vi "Receiver_Example - 2 Channel - Experiment_8.vi"() -> ()   [LabVIEW 2022 SP3]
uses:
  <vilib>/httpClient/LabVIEWHTTPClient.lvlib
panel:
  out "Boolean 7":bool
  out "HP - CH0":dbl format="%#_4g"
  out "Numeric":i32
  out "Boolean 6":bool
  out "Boolean 5":bool
  in  "url":string="http://Cobot280-01.local:5000"
  out "x = 0?":bool
  out "iterationsIM":dbl
  in  "State":i32
  in  "Counter":dbl
  in  "OFDM - 4QAM/16QAM":bool
  in  "Tab Control 3":enum32{"OFDM - 4QAM", "16QAM"}(tab)
  in  "Tab Control":enum32{"USRP Parameters", "Rx Info", "BER"}(tab)
  in  "USRP ControledParameters":T1={"Active Antenna"="RX2", "Gain (dB)"=10.0, "Carrier Frequency"=2400000000.0, "IQ Rate"=2000000.0, "Active channels"="0,1"} {"IQ Rate" format="%#_6p"; "Carrier Frequency" format="%#_6p"; "Gain (dB)" format="%#_6f"}
  in  "Device selection":refnum<k15>="RIO0"
  in  "Trigger level":dbl=0.005 format="%f"
  out "CH0":T2
  out "CH1":T2
  out "SIG valid? - CH1":bool
  out "SIG valid? - CH0":bool
  out "Frequency offset - CH1":dbl
  out "Frequency offset - CH0":dbl
  out "Coerced Parameters":T3={"IQ Rate"=100000.0, "Carrier  Freq."=100000.0, "Gain"=0.0} {"Gain" format="%#_6f"; "Carrier  Freq." format="%#_6p"; "IQ Rate" format="%#_6p"}
  out "Error out":errorcluster
  in  "Expected message LP - CH0":string="Non Critical Data\nNon Critical Data\nNon Critical Data\nNon Critical Data\nNon Critical Data"
  in  "Expected message - CH1":string="Critical Dataaaaa\nCritical Dataaaaa\nCritical Dataaaaa\nCritical Dataaaaa\nCritical Dataaaaa"
  out "Expected message LP Detected CH0":string="Non Critical Data\nNon Critical Data\nNon Critical Data\nNon Critical Data\nNon Critical Data"
  out "Expected message HP Detected CH1":string="Non Critical Data\nNon Critical Data\nNon Critical Data\nNon Critical Data\nNon Critical Data"
  in  "Boolean":bool
  in  "Boolean 3":bool
  out "Expected message HP Detected CH0":string="Non Critical Data\nNon Critical Data\nNon Critical Data\nNon Critical Data\nNon Critical Data"
  in  "Expected message HP - CH0":string="Critical Dataaaaa\nCritical Dataaaaa\nCritical Dataaaaa\nCritical Dataaaaa\nCritical Dataaaaa"
  in  "Boolean 2":bool
  out "Inst. BER HP - CH0":dbl format="%#_4g"
  out "Acc. BER HP - CH0":dbl format="%#_4g"
  out "Acum. Err HP - CH0":dbl
  out "No. Bits HP - CH0":dbl
  out "Acc. BER LP - CH0":dbl format="%#_4g"
  out "Inst. BER - CH1":dbl format="%#_4g"
  out "Inst. BER LP - CH0":dbl format="%#_4g"
  out "No. Bits - CH1":dbl
  out "No. Bits LP - CH0":dbl
  out "Acum. Err - CH1":dbl
  out "Acum. Err LP - CH0":dbl
  in  "Record BER":bool
  in  "Refresh Button":bool
  out "Acc. BER - CH1":dbl format="%#_4g"
  in  "Low-Power Window Size - CH0":dbl=15.0 format="%#_6p"
  in  "High-Power Window Size":dbl=15.0 format="%#_6p"
  in  "Tab Control 2":enum32{"1 Channel", "2 Channel"}(tab)
  in  "Save data 1 channel":bool
  out "Constellation Map 1 Channel":cdb[](graph)
  out "Low-Power BER - 1 Channel":dbl(graph)
  out "High-Power BER - 1 Channel":dbl(graph)
  out "High-Power Decoded message - 1 Channel":string
  out "Low-Power Decoded message - 1 Channel":string
  out "Low-Power Decoded message - CH0":string
  out "Decoded message - CH1":string
  out "Constellation Map 2 Channel":cluster{"Constellation":cdb[]}[](graph)
  out "Low-Power BER - CH0":dbl(graph)
  out "High-Power BER":T4(graph)
  out "High-Power Decoded message - CH0":string
  out "CH1 2":bool
  out "CH0 2":bool
  in  "Save data 2 channels":bool
  in  "Channel":bool
  in  "Save data":bool
  out "Expected message  HP  Detected 2":string="Critical Dataaaaa\nCritical Dataaaaa\nCritical Dataaaaa\nCritical Dataaaaa\nCritical Dataaaaa"
  in  "Boolean 4":bool
  in  "High-Power Window Size 2":dbl=15.0 format="%#_6p"
  out "High-Power Instantaneous BER Graph 2":u8(slide) scale=0.0..100.0
  out "High-Power BER Graph 2":dbl(graph)
  out "No. Bits HP 2":dbl
  out "Acc. BER  HP 2":dbl format="%#_4g"
  out "Acum. Err HP 2":dbl
  out "Inst. BER HP 2":dbl format="%#_4g"
  in  "Expected message 2 HP 2":string="Critical Dataaaaa\nCritical Dataaaaa\nCritical Dataaaaa\nCritical Dataaaaa\nCritical Dataaaaa"
  out "High-Power Decoded Message 2":string
  in  "Record BER 2":bool
  out "Constellation Map 2":cdb[](graph)
  out "Frequency offset 2":dbl
  out "SIG valid? 2":bool
  in  "Refresh Button 2":bool
  out "Error out 2":errorcluster
  in  "error in (no error)":errorcluster
  # "OFDM Superposition Coded Receiver"
  # "1 Channel"
  # "2 Channel"
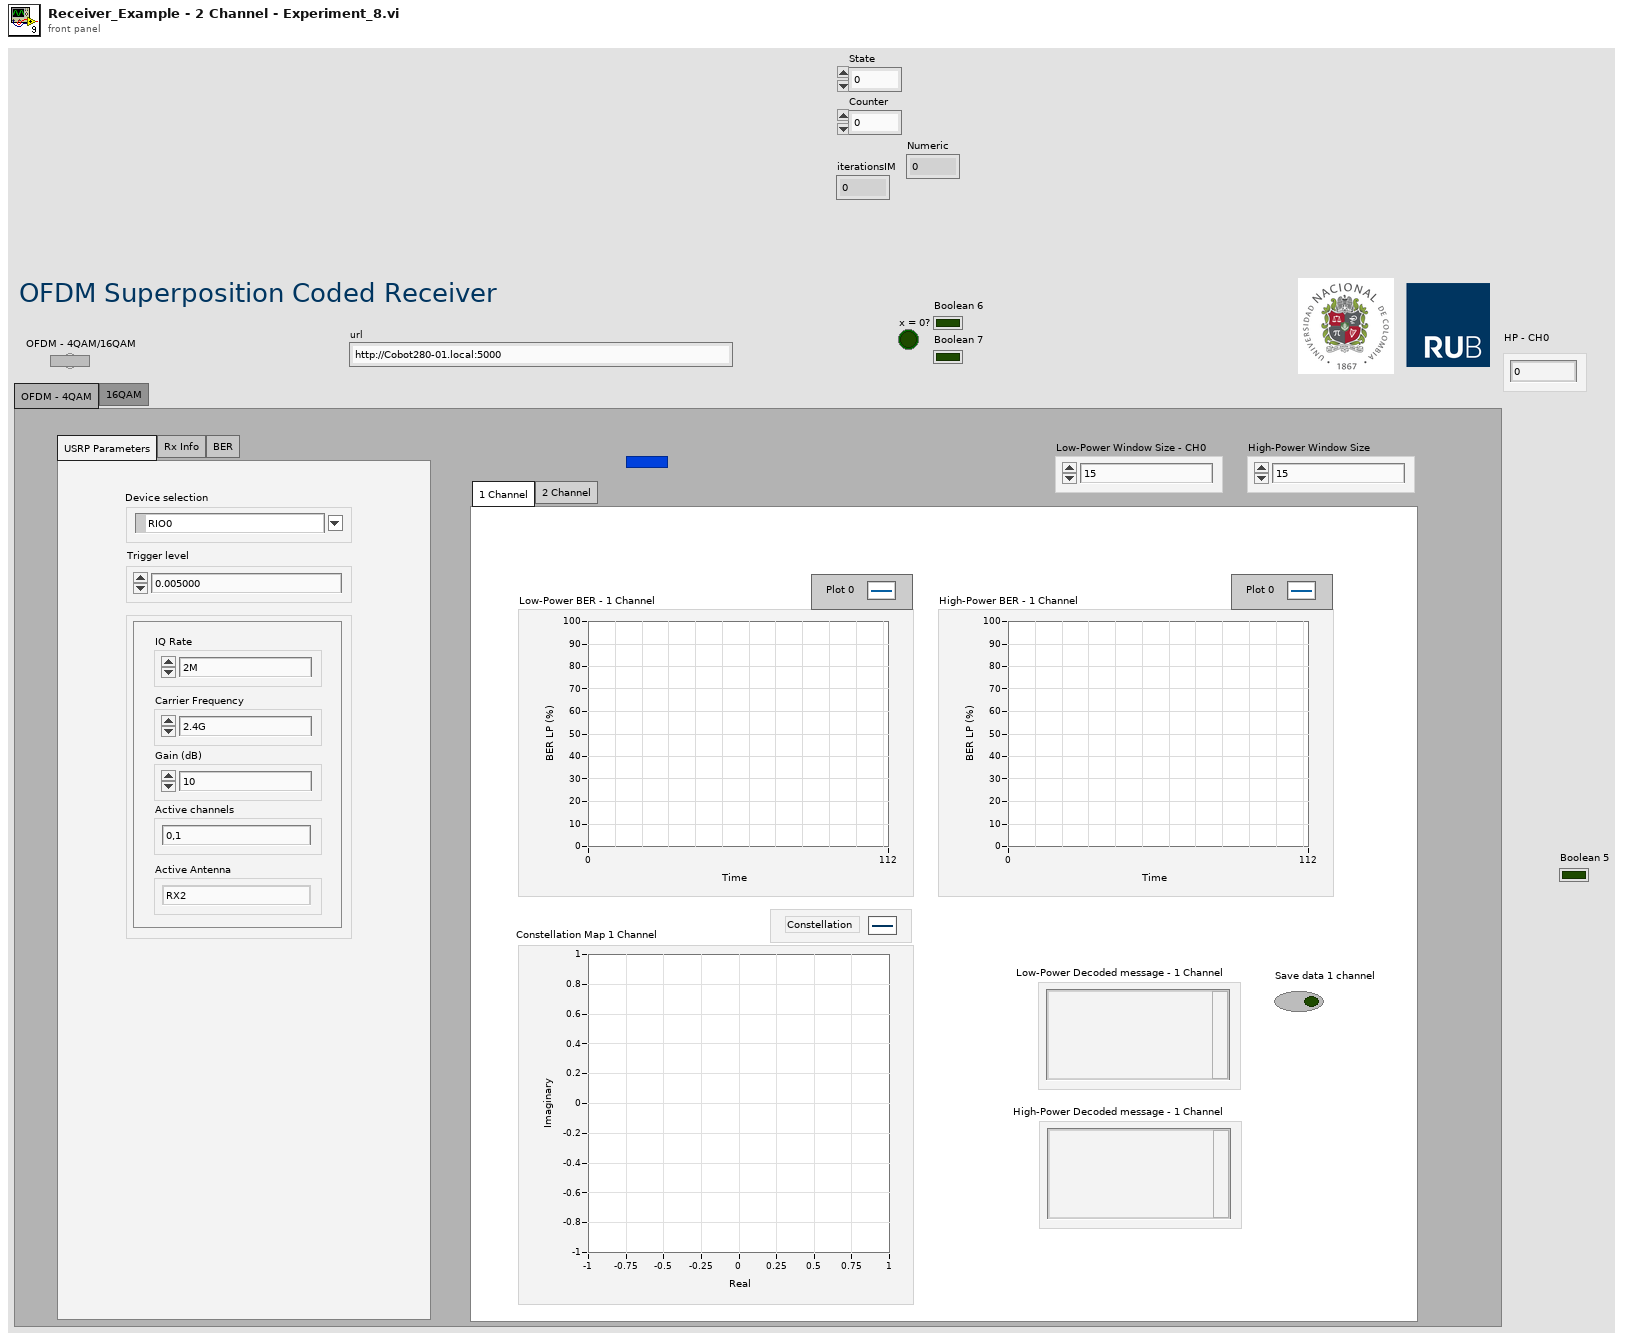
[diagram p1: front panel]
types:
  T1 = cluster{"Active Antenna":string, "Gain (dB)":dbl, "Carrier Frequency":dbl, "IQ Rate":dbl, "Active channels":string}
  T2 = cluster{"Modulation type":enum16{"QPSK(4QAM)", "64QAM", "16QAM", "BPSK"}, "BCC rate (k/n)":enum16{"1/2", "2/3", "3/4"}}
  T3 = cluster{"IQ Rate":dbl, "Carrier  Freq.":dbl, "Gain":dbl}
  T4 = cluster{"Graph Instantaneous BER":dbl, "Graph Instantaneous BER":dbl, "Inst. BER - CH1":dbl}
  T5 = enum16{"open", "replace", "create", "open or create", "replace or create", "replace or create with confirmation"}
  T6 = typedef "LabVIEWHTTPClient.lvlib/ClientHandle.ctl" = refnum<k1>
  T7 = typedef "angle_speed_def.ctl" = cluster{"degrees":dbl[], "speed":i32}
  T8 = cluster{"coerced IQ rate":dbl, "coerced carrier frequency":dbl, "coerced gain":dbl}
  T9 = cluster{"Graph Instantaneous BER":dbl, "Graph Instantaneous BER":dbl, "Graph Instantaneous BER":dbl}
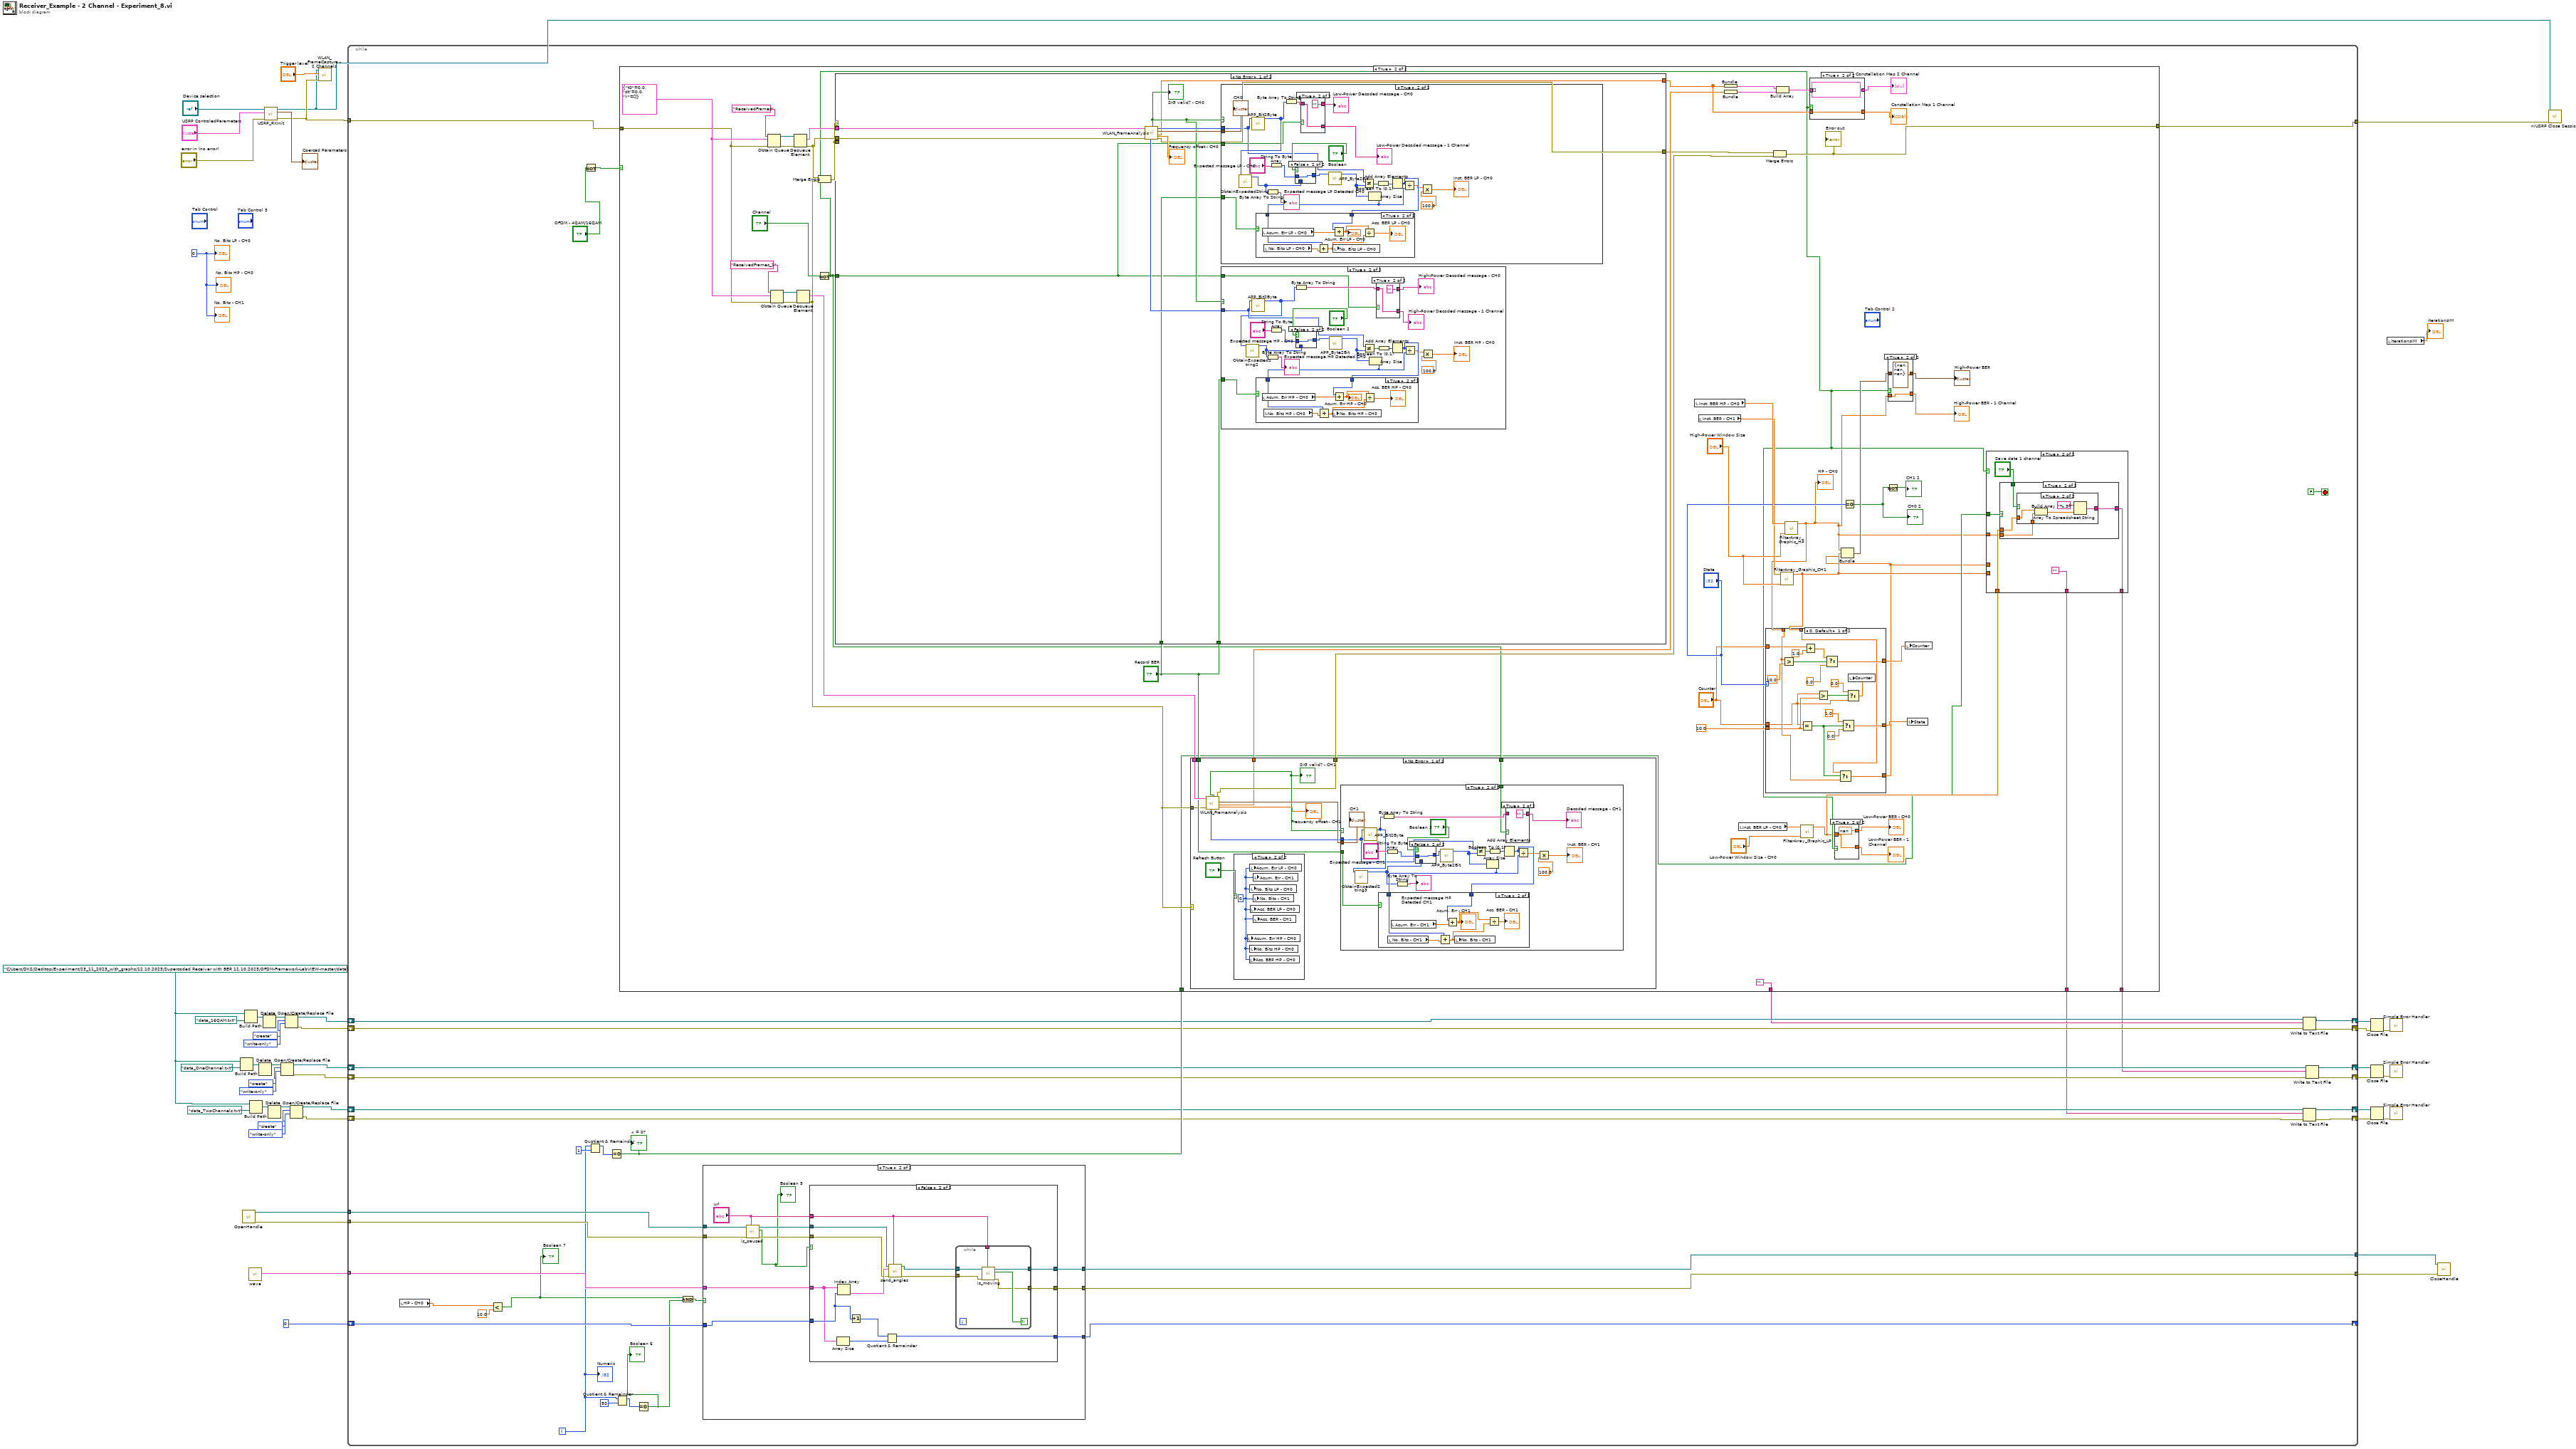
[diagram p0: block diagram]
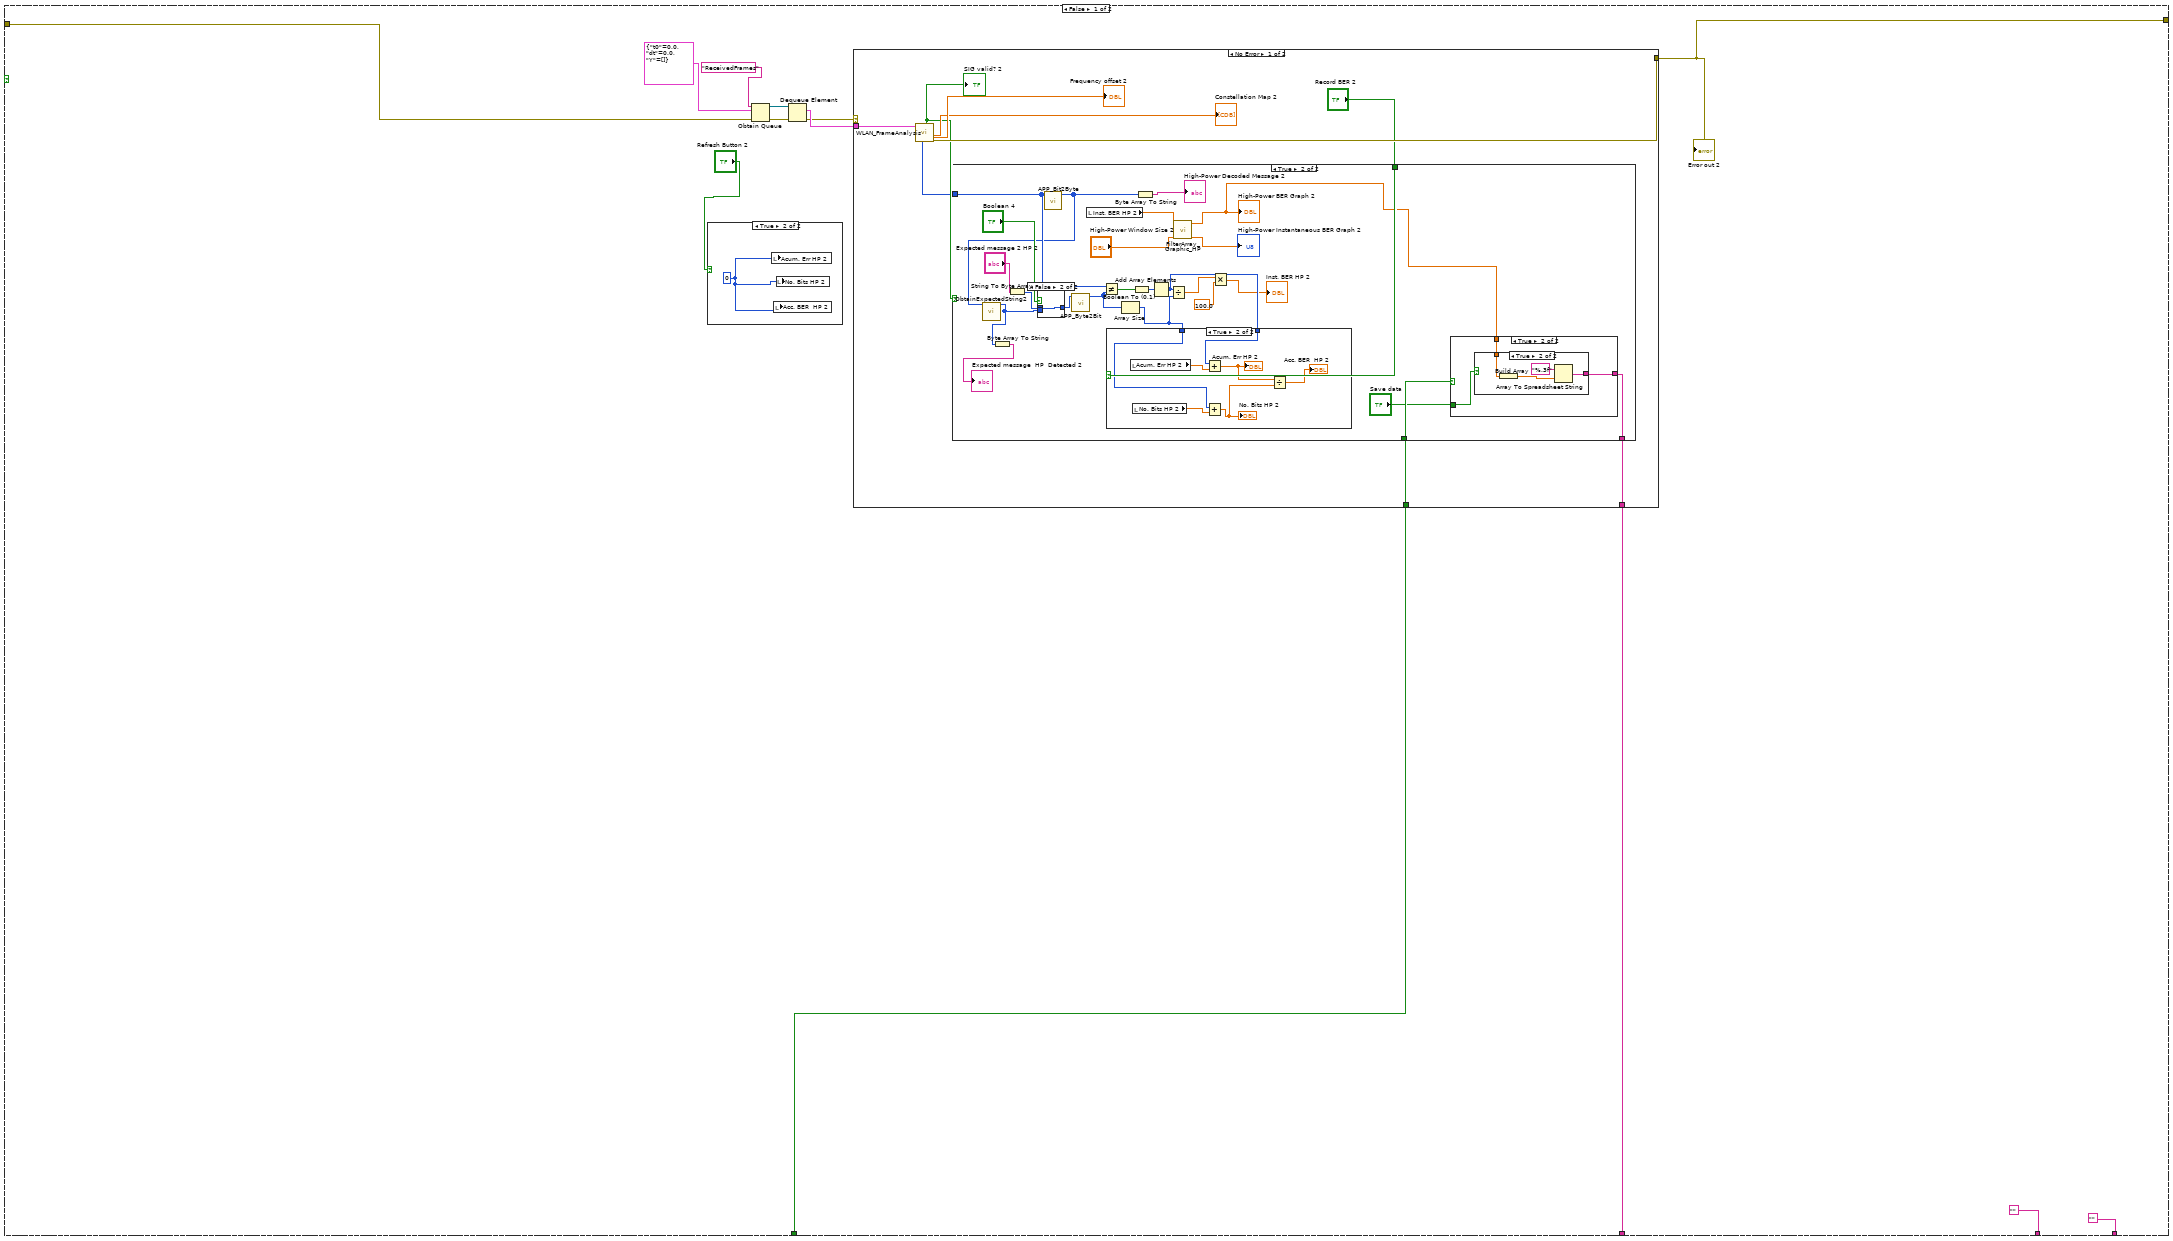
[diagram p4: hidden frame]
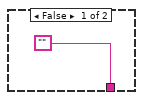
[diagram p6: hidden frame]
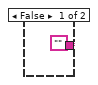
[diagram p7: hidden frame]
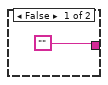
[diagram p8: hidden frame]
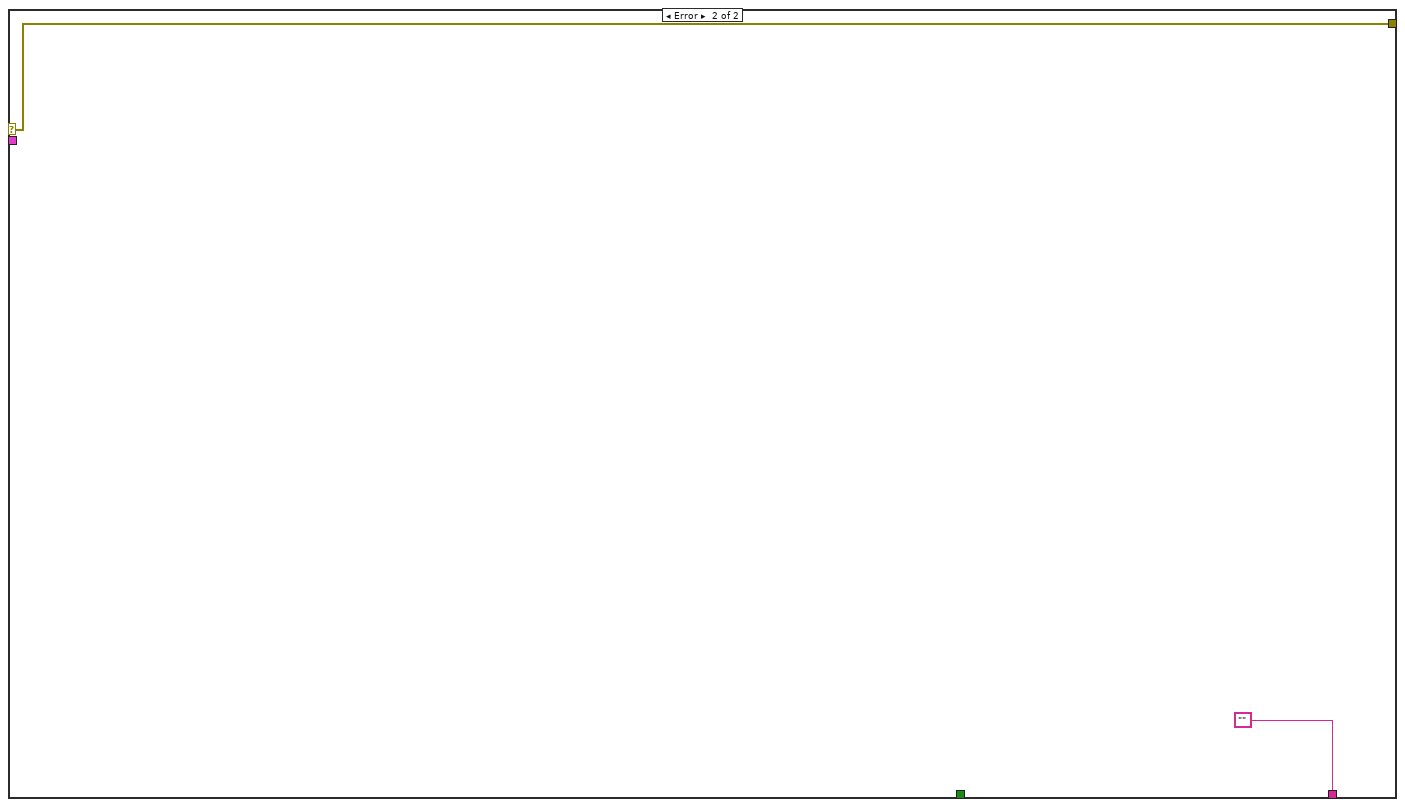
[diagram p11: hidden frame]
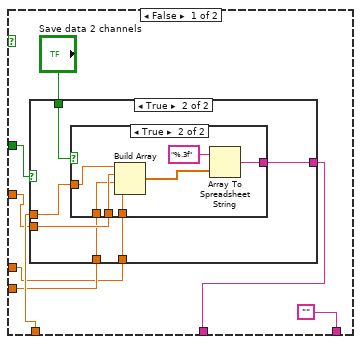
[diagram p12: hidden frame]
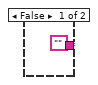
[diagram p13: hidden frame]
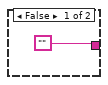
[diagram p14: hidden frame]
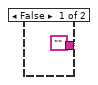
[diagram p15: hidden frame]
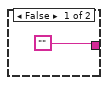
[diagram p16: hidden frame]
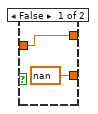
[diagram p17: hidden frame]
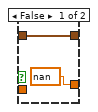
[diagram p18: hidden frame]
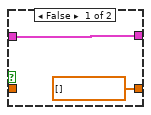
[diagram p19: hidden frame]
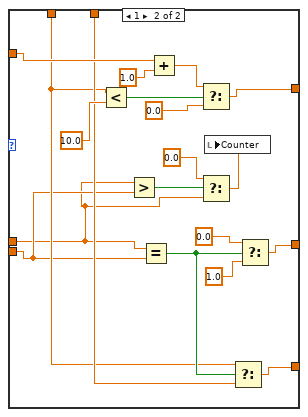
[diagram p20: hidden frame]
diagram:
  w17 = path "C:/Users/DKS/Desktop/Experiment/23_11_2023_with_graphs/12.10.2023/Supercoded Receiver with BER 12.10.2023/OFDM-Framework-LabVIEW-master/data"
  w39 = 0
  n1 = Build Path(base path=w17, name or relative path=path "data_OneChannel.txt" ("default name")) -> (appended path=w27:path)
  n2 = call <vilib>:"OpenHandle.vi"() -> ("client handle out"=w6:T6, "error out"=w5:errorcluster)  [unwired: 14 in]
  n3 = Build Path(base path=w17, name or relative path=path "data_16QAM.txt" ("default name")) -> (appended path=w37:path)
  n4 = call "wave.vi"() -> ("sequenz"=w4:T7[])  [unwired: 11 in]
  n5 = Build Path(base path=w17, name or relative path=path "data_TwoChannels.txt" ("default name")) -> (appended path=w22:path)
  n6 = Delete(path (use dialog)=w27) -> (deleted path=w26:path)  [unwired: 4 in, 2 out]
  n7 = Delete(path (use dialog)=w37) -> (deleted path=w36:path)  [unwired: 4 in, 2 out]
  n8 = call "USRP_RXInit.vi"("device names"="Device selection", "USRP ControledParameters"="USRP ControledParameters", "error in (no error)"="error in (no error)") -> ("session handle out"=w42:refnum<k15>, "USRP CoercedParamters"=→"Coerced Parameters":T8, "error out"=w45:errorcluster)  [unwired: 5 in]
  n9 = Delete(path (use dialog)=w22) -> (deleted path=w21:path)  [unwired: 4 in, 2 out]
  n10 = Open/Create/Replace File(file path (use dialog)=w26, operation (0:open)=T5."create", access (0:read/write)=enum16{"read/write", "read-only", "write-only"}."write-only") -> (refnum out=w14:refnum<file>, error out=w13:errorcluster)  [unwired: 1 in, 3 out]
  n11 = Open/Create/Replace File(file path (use dialog)=w36, operation (0:open)=T5."create", access (0:read/write)=enum16{"read/write", "read-only", "write-only"}."write-only") -> (refnum out=w30:refnum<file>, error out=w31:errorcluster)  [unwired: 1 in, 3 out]
  n12 = Open/Create/Replace File(file path (use dialog)=w21, operation (0:open)=T5."create", access (0:read/write)=enum16{"read/write", "read-only", "write-only"}."write-only") -> (refnum out=w12:refnum<file>, error out=w11:errorcluster)  [unwired: 1 in, 3 out]
  n13 = call "WLAN_FrameCapture - 2 Channels.vi"("error in (no error)"=w45, "Trigger level"="Trigger level", "session handle"=w42) -> ()  [unwired: 8 in]
  n14 = while {
    tunnel: w45 -> [w85]
    tunnel: [w84] -> w43
    shift-right: [w77] -> w29
    shift-left: w31 -> [w75]
    shift-right: [w76] -> w28
    shift-left: w30 -> [w74]
    shift-right: [w71] -> w10
    shift-left: w14 -> [w72]
    shift-right: [w69] -> w9
    shift-left: w13 -> [w70]
    shift-right: [w65] -> w8
    shift-left: w12 -> [w68]
    shift-right: [w66] -> w7
    shift-left: w11 -> [w67]
    tunnel: w6 -> [w59]
    tunnel: w5 -> [w60]
    tunnel: w4 -> [w62]
    shift-right: [w58] -> _
    shift-left: 0 -> [w61]
    tunnel: [w57] -> w2
    tunnel: [w56] -> w1
    i -> [w53]
    stop <- FALSE stop-if-true
    n15 = local read "HP - CH0"() -> (w50:dbl)
    n16 = Less?(x=w50, y=10.0) -> (x < y?=w48:bool)
    "Boolean 7" <- w48
    n17 = Not(x="OFDM - 4QAM/16QAM") -> (.not. x?=w82:bool)
    n18 = Quotient & Remainder(x=w53, y=1) -> (x-y*floor(x/y)=w79:i32)  [unwired: 1 out]
    n19 = Equal To 0?(x=w79) -> (x = 0?=w78:bool)
    "x = 0?" <- w78
    n20 = Quotient & Remainder(x=w53, y=50) -> (x-y*floor(x/y)=w54:i32)  [unwired: 1 out]
    n21 = case shown="True" w82 {
      tunnel: w85 -> [w127 w205]
      tunnel: [w126 w204] -> w84
      tunnel: w78 -> [w125 w196]
      tunnel: [w124 ""] -> w73
      tunnel: ["" w195] -> w64
      tunnel: ["" w193] -> w63
      frame False {
        n22 = case shown="True" "Refresh Button 2" {
          frame False {
          }
          frame True {
            w135 = 0
            n23 = local write "Acum. Err HP 2"(w135) -> ()
            n24 = local write "Acc. BER  HP 2"(w135) -> ()
            n25 = local write "No. Bits HP 2"(w135) -> ()
          }
        }
        n26 = Obtain Queue(name (unnamed)="ReceivedFrames", element data type=cluster{"t0":dbl, "dt":dbl, "Y":cdb[]} {"t0"=0.0, "dt"=0.0, "Y"=[]} ("data"), error in (no error)=w127) -> (queue out=w128:refnum<queue>, error out=w131:errorcluster)  [unwired: 2 in, 1 out]
        n27 = Dequeue Element(queue=w128, error in (no error)=w131) -> (element=w130:cluster{"t0":dbl, "dt":dbl, "Y":cdb[]}, error out=w129:errorcluster)  [unwired: 1 in, 2 out]
        n28 = case shown="No Error" w129 {
          selector: w129 -> [_ w190]
          tunnel: w130 -> [w143 _]
          tunnel: [w144 w190] -> w126
          tunnel: w125 -> [w137 _]
          tunnel: [w136 ""] -> w124
          frame No Error {
            n29 = call "WLAN_FrameAnalysis.vi"("input cluster"=w143) -> ("error out"=w144:errorcluster, "Constellation"=→"Constellation Map 2":cdb[], "Frequency offset"=→"Frequency offset 2":dbl, "SIG valid?"=w139:bool, "outputbitsHP"=w138:i8[])  [unwired: 4 in, 2 out]
            "SIG valid? 2" <- w139
            n30 = case shown="True" w139 {
              tunnel: "Record BER 2" -> [_ w164]
              tunnel: w138 -> [_ w159]
              tunnel: w137 -> [_ w148]
              tunnel: ["" w146] -> w136
              frame False {
              }
              frame True {
                n31 = String To Byte Array(string="Expected message 2 HP 2") -> (unsigned byte array=w157:u8[])
                n32 = call "APP_Bit2Byte.vi"("input bit stream"=w159) -> ("output byte stream"=w153:u8[])  [unwired: 10 in]
                n33 = call "ObtainExpectedString2.vi"("Array"=w153) -> ("detectedMessage"=w155:i8[])  [unwired: 9 in]
                n34 = Byte Array To String(unsigned byte array=w155) -> (string=→"Expected message  HP  Detected 2":string)
                n35 = case shown="False" "Boolean 4" {
                  tunnel: [w180 w181] -> w158
                  tunnel: w157 -> [_ w181]
                  tunnel: w155 -> [w180 _]
                  frame True {
                  }
                  frame False {
                  }
                }
                n36 = call "APP_Byte2Bit.vi"("input byte stream"=w158) -> ("output bit stream"=w160:i8[])  [unwired: 10 in]
                n37 = local read "Inst. BER HP 2"() -> (w163:dbl)
                n38 = Not Equal?(x=w159, y=w160) -> (x != y?=w168:bool[])
                n39 = Array Size(array=w160) -> (size(s)=w165:i32)
                n40 = Boolean To (0,1)(Boolean=w168) -> (0, 1=w167:i16[])
                n41 = Byte Array To String(unsigned byte array=w153) -> (string=→"High-Power Decoded Message 2":string)
                n42 = Add Array Elements(numeric array=w167) -> (sum=w166:i16)
                n43 = case shown="True" w164 {
                  tunnel: w166 -> [_ w187]
                  tunnel: w165 -> [_ w182]
                  frame False {
                  }
                  frame True {
                    n44 = local read "Acum. Err HP 2"() -> (w188:dbl)
                    n45 = local read "No. Bits HP 2"() -> (w184:dbl)
                    n46 = Add(x=w187, y=w188) -> (x+y=w186:dbl)
                    "Acum. Err HP 2" <- w186
                    n47 = Add(x=w182, y=w184) -> (x+y=w183:dbl)
                    "No. Bits HP 2" <- w183
                    n48 = Divide(x=w186, y=w183) -> (x/y=→"Acc. BER  HP 2":dbl)
                  }
                }
                n49 = Divide(x=w166, y=w165) -> (x/y=w152:dbl)
                n50 = call "FilterArray_Graphic_HP.vi"("Window Size"="High-Power Window Size 2", "Instantaneous BER"=w163) -> ("Slide Bar"=→"High-Power Instantaneous BER Graph 2":dbl, "Graph Instantaneous BER"=w149:dbl)  [unwired: 4 in]
                "High-Power BER Graph 2" <- w149
                n51 = Multiply(x=w152, y=100.0) -> (x*y=→"Inst. BER HP 2":dbl)
                n52 = case shown="True" w148 {
                  tunnel: ["" w174] -> w146
                  tunnel: w149 -> [_ w173]
                  tunnel: "Save data" -> [_ w172]
                  frame False {
                  }
                  frame True {
                    n53 = case shown="True" w172 {
                      tunnel: ["" w177] -> w174
                      tunnel: w173 -> [_ w176]
                      frame False {
                      }
                      frame True {
                        n54 = Build Array(w176) -> (w179:dbl[])
                        n55 = Array To Spreadsheet String(array=w179, 3:"%.3f") -> (spreadsheet string=w177:string)  [unwired: 1 out]
                      }
                    }
                  }
                }
              }
            }
          }
          frame Error {
          }
        }
        "Error out 2" <- w126
      }
      frame True {
        w241 = cluster{"t0":dbl, "dt":dbl, "Y":cdb[]} {"t0"=0.0, "dt"=0.0, "Y"=[]} ("data")
        n56 = Obtain Queue(name (unnamed)="ReceivedFrames", element data type=w241, error in (no error)=w205) -> (queue out=w206:refnum<queue>, error out=w208:errorcluster)  [unwired: 2 in, 1 out]
        n57 = Obtain Queue(name (unnamed)="ReceivedFrames_1", element data type=w241, error in (no error)=w205) -> (queue out=w210:refnum<queue>, error out=w211:errorcluster)  [unwired: 2 in, 1 out]
        n58 = Dequeue Element(queue=w206, error in (no error)=w208) -> (element=w207:cluster{"t0":dbl, "dt":dbl, "Y":cdb[]}, error out=w214:errorcluster)  [unwired: 1 in, 2 out]
        n59 = Dequeue Element(queue=w210, error in (no error)=w211) -> (element=w216:cluster{"t0":dbl, "dt":dbl, "Y":cdb[]}, error out=w220:errorcluster)  [unwired: 1 in, 2 out]
        n60 = Not(x="Channel") -> (.not. x?=w198:bool)
        n61 = Merge Errors(w214, w220) -> (w213:errorcluster)
        n62 = case shown="No Error" w213 {
          tunnel: w207 -> [w386 _]
          tunnel: w213 -> [_ w460]
          tunnel: w214 -> [w383 _]
          tunnel: [w382 dbl[] []] -> w232
          tunnel: [w381 w460] -> w217
          tunnel: "Record BER" -> [w380 _]
          tunnel: "Record BER" -> [w379 _]
          tunnel: w198 -> [w378 _]
          frame No Error {
            n63 = call "WLAN_FrameAnalysis.vi"("error in (no error)"=w383, "input cluster"=w386) -> ("error out"=w381:errorcluster, "Constellation"=w382:cdb[], "Modulation parameter"=w387:T2, "output bits"=w388:i8[], "Frequency offset"=→"Frequency offset - CH0":dbl, "SIG valid?"=w384:bool, "outputbitsHP"=w385:i8[])  [unwired: 3 in]
            "SIG valid? - CH0" <- w384
            n64 = case shown="True" w384 {
              tunnel: w388 -> [_ w429]
              tunnel: w387 -> [_ w445]
              tunnel: w379 -> [_ w441]
              tunnel: w378 -> [_ w424]
              frame False {
              }
              frame True {
                n65 = call "APP_Bit2Byte.vi"("input bit stream"=w429) -> ("output byte stream"=w433:u8[])  [unwired: 10 in]
                n66 = call "ObtainExpectedString.vi"("Array"=w433) -> ("detectedMessage"=w430:i8[])  [unwired: 9 in]
                n67 = Byte Array To String(unsigned byte array=w430) -> (string=→"Expected message LP Detected CH0":string)
                n68 = String To Byte Array(string="Expected message LP - CH0") -> (unsigned byte array=w434:u8[])
                n69 = Byte Array To String(unsigned byte array=w433) -> (string=w427:string)
                n70 = case shown="False" "Boolean" {
                  tunnel: [w450 w451] -> w436
                  tunnel: w434 -> [_ w451]
                  tunnel: w430 -> [w450 _]
                  frame True {
                  }
                  frame False {
                  }
                }
                n71 = case shown="True" w424 {
                  tunnel: w427 -> [w447 w449]
                  tunnel: ["" ("string") w449] -> w426
                  tunnel: [w447 "" ("string")] -> w425
                  frame False {
                  }
                  frame True {
                  }
                }
                "Low-Power Decoded message - CH0" <- w425
                "Low-Power Decoded message - 1 Channel" <- w426
                n72 = call "APP_Byte2Bit.vi"("input byte stream"=w436) -> ("output bit stream"=w435:i8[])  [unwired: 10 in]
                n73 = Not Equal?(x=w429, y=w435) -> (x != y?=w443:bool[])
                n74 = Array Size(array=w435) -> (size(s)=w440:i32)
                n75 = Boolean To (0,1)(Boolean=w443) -> (0, 1=w444:i16[])
                n76 = Add Array Elements(numeric array=w444) -> (sum=w439:i16)
                n77 = case shown="True" w441 {
                  tunnel: w440 -> [_ w457]
                  tunnel: w439 -> [_ w455]
                  frame False {
                  }
                  frame True {
                    n78 = local read "Acum. Err LP - CH0"() -> (w456:dbl)
                    n79 = local read "No. Bits LP - CH0"() -> (w458:dbl)
                    n80 = Add(x=w457, y=w458) -> (x+y=w454:dbl)
                    n81 = Add(x=w455, y=w456) -> (x+y=w453:dbl)
                    "Acum. Err LP - CH0" <- w453
                    n82 = local write "No. Bits LP - CH0"(w454) -> ()
                    n83 = Divide(x=w453, y=w454) -> (x/y=→"Acc. BER LP - CH0":dbl)
                  }
                }
                n84 = Divide(x=w439, y=w440) -> (x/y=w438:dbl)
                n85 = Multiply(x=w438, y=100.0) -> (x*y=→"Inst. BER LP - CH0":dbl)
                "CH0" <- w445
              }
            }
            n86 = case shown="True" w384 {
              tunnel: w385 -> [_ w397]
              tunnel: w380 -> [_ w407]
              tunnel: w378 -> [_ w390]
              frame False {
              }
              frame True {
                n87 = call "APP_Bit2Byte.vi"("input bit stream"=w397) -> ("output byte stream"=w396:u8[])  [unwired: 10 in]
                n88 = call "ObtainExpectedString2.vi"("Array"=w396) -> ("detectedMessage"=w395:i8[])  [unwired: 9 in]
                n89 = Byte Array To String(unsigned byte array=w395) -> (string=→"Expected message HP Detected CH0":string)
                n90 = String To Byte Array(string="Expected message HP - CH0") -> (unsigned byte array=w400:u8[])
                n91 = Byte Array To String(unsigned byte array=w396) -> (string=w391:string)
                n92 = case shown="False" "Boolean 2" {
                  tunnel: [w415 w416] -> w402
                  tunnel: w400 -> [_ w416]
                  tunnel: w395 -> [w415 _]
                  frame True {
                  }
                  frame False {
                  }
                }
                n93 = call "APP_Byte2Bit.vi"("input byte stream"=w402) -> ("output bit stream"=w401:i8[])  [unwired: 10 in]
                n94 = Not Equal?(x=w397, y=w401) -> (x != y?=w409:bool[])
                n95 = Array Size(array=w401) -> (size(s)=w406:i32)
                n96 = case shown="True" w390 {
                  tunnel: w391 -> [w412 w414]
                  tunnel: ["" ("string") w414] -> w392
                  tunnel: [w412 "" ("string")] -> w393
                  frame False {
                  }
                  frame True {
                  }
                }
                "High-Power Decoded message - CH0" <- w393
                "High-Power Decoded message - 1 Channel" <- w392
                n97 = Boolean To (0,1)(Boolean=w409) -> (0, 1=w410:i16[])
                n98 = Add Array Elements(numeric array=w410) -> (sum=w405:i16)
                n99 = case shown="True" w407 {
                  tunnel: w406 -> [_ w422]
                  tunnel: w405 -> [_ w420]
                  frame False {
                  }
                  frame True {
                    n100 = local read "Acum. Err HP - CH0"() -> (w421:dbl)
                    n101 = local read "No. Bits HP - CH0"() -> (w423:dbl)
                    n102 = Add(x=w422, y=w423) -> (x+y=w419:dbl)
                    n103 = local write "No. Bits HP - CH0"(w419) -> ()
                    n104 = Add(x=w420, y=w421) -> (x+y=w418:dbl)
                    "Acum. Err HP - CH0" <- w418
                    n105 = Divide(x=w418, y=w419) -> (x/y=→"Acc. BER HP - CH0":dbl)
                  }
                }
                n106 = Divide(x=w405, y=w406) -> (x/y=w404:dbl)
                n107 = Multiply(x=w404, y=100.0) -> (x*y=→"Inst. BER HP - CH0":dbl)
              }
            }
          }
          frame Error {
          }
        }
        n108 = case shown="No Error" w220 {
          tunnel: w216 -> [w338 _]
          tunnel: "Record BER" -> [w336 _]
          tunnel: [w335 w377] -> w218
          tunnel: [w334 dbl[] []] -> w219
          tunnel: w220 -> [w333 w377]
          tunnel: w198 -> [w332 _]
          frame No Error {
            n109 = call "WLAN_FrameAnalysis.vi"("error in (no error)"=w333, "input cluster"=w338) -> ("error out"=w335:errorcluster, "Constellation"=w334:cdb[], "Modulation parameter"=w341:T2, "Frequency offset"=→"Frequency offset - CH1":dbl, "SIG valid?"=w337:bool, "outputbitsHP"=w339:i8[])  [unwired: 3 in, 1 out]
            "SIG valid? - CH1" <- w337
            n110 = case shown="True" "Refresh Button" {
              frame False {
              }
              frame True {
                w343 = 0
                n111 = local write "Acum. Err HP - CH0"(w343) -> ()
                n112 = local write "Acc. BER HP - CH0"(w343) -> ()
                n113 = local write "Acum. Err LP - CH0"(w343) -> ()
                n114 = local write "No. Bits LP - CH0"(w343) -> ()
                n115 = local write "No. Bits HP - CH0"(w343) -> ()
                n116 = local write "Acc. BER LP - CH0"(w343) -> ()
                n117 = local write "Acum. Err - CH1"(w343) -> ()
                n118 = local write "No. Bits - CH1"(w343) -> ()
                n119 = local write "Acc. BER - CH1"(w343) -> ()
              }
            }
            n120 = case shown="True" w337 {
              tunnel: w339 -> [_ w350]
              tunnel: w341 -> [_ w364]
              tunnel: w336 -> [_ w347]
              tunnel: w332 -> [_ w344]
              frame False {
              }
              frame True {
                n121 = call "APP_Bit2Byte.vi"("input bit stream"=w350) -> ("output byte stream"=w353:u8[])  [unwired: 10 in]
                n122 = call "ObtainExpectedString3.vi"("Array"=w353) -> ("detectedMessage"=w352:i8[])  [unwired: 9 in]
                n123 = Byte Array To String(unsigned byte array=w353) -> (string=w345:string)
                n124 = String To Byte Array(string="Expected message - CH1") -> (unsigned byte array=w354:u8[])
                n125 = Byte Array To String(unsigned byte array=w352) -> (string=→"Expected message HP Detected CH1":string)
                n126 = case shown="False" "Boolean 3" {
                  tunnel: [w367 w368] -> w356
                  tunnel: w354 -> [_ w368]
                  tunnel: w352 -> [w367 _]
                  frame True {
                  }
                  frame False {
                  }
                }
                n127 = call "APP_Byte2Bit.vi"("input byte stream"=w356) -> ("output bit stream"=w355:i8[])  [unwired: 10 in]
                n128 = Not Equal?(x=w350, y=w355) -> (x != y?=w362:bool[])
                n129 = Array Size(array=w355) -> (size(s)=w360:i32)
                n130 = Boolean To (0,1)(Boolean=w362) -> (0, 1=w363:i16[])
                n131 = Add Array Elements(numeric array=w363) -> (sum=w359:i16)
                n132 = case shown="True" w347 {
                  tunnel: w360 -> [_ w374]
                  tunnel: w359 -> [_ w372]
                  frame False {
                  }
                  frame True {
                    n133 = local read "No. Bits - CH1"() -> (w375:dbl)
                    n134 = local read "Acum. Err - CH1"() -> (w373:dbl)
                    n135 = Add(x=w374, y=w375) -> (x+y=w371:dbl)
                    n136 = Add(x=w372, y=w373) -> (x+y=w370:dbl)
                    "Acum. Err - CH1" <- w370
                    n137 = local write "No. Bits - CH1"(w371) -> ()
                    n138 = Divide(x=w370, y=w371) -> (x/y=→"Acc. BER - CH1":dbl)
                  }
                }
                n139 = case shown="True" w344 {
                  tunnel: w345 -> [w365 _]
                  tunnel: [w365 "" ("string")] -> w346
                  frame False {
                  }
                  frame True {
                  }
                }
                "Decoded message - CH1" <- w346
                n140 = Divide(x=w359, y=w360) -> (x/y=w357:dbl)
                n141 = Multiply(x=w357, y=100.0) -> (x*y=→"Inst. BER - CH1":dbl)
                "CH1" <- w364
              }
            }
          }
          frame Error {
          }
        }
        n142 = local read "Inst. BER HP - CH0"() -> (w237:dbl)
        n143 = local read "Inst. BER - CH1"() -> (w227:dbl)
        n144 = Bundle("Constellation"=w232) -> (w231:cluster{"Constellation":cdb[]})  [unwired: 1 in]
        n145 = Bundle("Constellation"=w219) -> (w215:cluster{"Constellation":cdb[]})  [unwired: 1 in]
        n146 = local read "Inst. BER LP - CH0"() -> (w200:dbl)
        n147 = Merge Errors(w217, w218) -> (w204:errorcluster)
        "Error out" <- w204
        n148 = Build Array(w231, w215) -> (w234:cluster{"Constellation":cdb[]}[])
        n149 = call "FilterArray_Graphic_CH1.vi"("Window Size"="High-Power Window Size", "Instantaneous BER"=w227) -> ("Graph Instantaneous BER"=w194:dbl)  [unwired: 4 in, 1 out]
        n150 = call "FilterArray_Graphic_HP.vi"("Window Size"="High-Power Window Size", "Instantaneous BER"=w237) -> ("Graph Instantaneous BER"=w191:dbl)  [unwired: 4 in, 1 out]
        "HP - CH0" <- w191
        n151 = case shown="0, Default" "State" {
          tunnel: "Counter" -> [w300 w320]
          tunnel: [w307 w323] -> w223
          tunnel: "Counter" -> [w295 w313]
          tunnel: [w304 w322] -> w224
          tunnel: [w302 w321] -> w192
          tunnel: w191 -> [w301 w318]
          tunnel: w194 -> [w299 w319]
          tunnel: 10.0 ("y") -> [w298 w314]
          frame 0, Default {
            n152 = Greater?(x=w301, y=10.0) -> (0:w308:bool)
            n153 = Equal?(x=w295, y=w298) -> (x = y?=w303:bool)
            n154 = Add(x=w300, y=1.0) -> (x+y=w310:dbl)
            n155 = Greater?(x=w295, y=w298) -> (0:w297:bool)
            n156 = Select(t=w310, s=w308, f=0.0) -> (s? t:f=w307:dbl)
            n157 = Select(t=w299, s=w303, f=w301) -> (s? t:f=w302:dbl)
            n158 = Select(t=1.0, s=w303, f=0.0) -> (s? t:f=w304:dbl)
            n159 = Select(t=0.0, s=w297, f=w295) -> (s? t:f=w294:dbl)
            n160 = local write "Counter"(w294) -> ()
          }
          frame 1 {
            n161 = Less?(x=w318, y=10.0) -> (x < y?=w324:bool)
            n162 = Greater?(x=w313, y=w314) -> (0:w316:bool)
            n163 = Equal?(x=w313, y=w314) -> (x = y?=w326:bool)
            n164 = Add(x=w320, y=1.0) -> (x+y=w330:dbl)
            n165 = Select(t=w330, s=w324, f=0.0) -> (s? t:f=w323:dbl)
            n166 = Select(t=0.0, s=w316, f=w313) -> (s? t:f=w317:dbl)
            n167 = local write "Counter"(w317) -> ()
            n168 = Select(t=w318, s=w326, f=w319) -> (s? t:f=w321:dbl)
            n169 = Select(t=0.0, s=w326, f=1.0) -> (s? t:f=w322:dbl)
          }
        }
        n170 = call "FilterArray_Graphic_LP.vi"("Window Size"="Low-Power Window Size - CH0", "Instantaneous BER"=w200) -> ("Graph Instantaneous BER"=w197:dbl)  [unwired: 4 in, 1 out]
        n171 = case shown="True" w198 {
          tunnel: [cdb[] [] ("Constellation") w293] -> w233
          tunnel: w232 -> [_ w293]
          tunnel: w234 -> [w291 _]
          tunnel: [w291 cluster{"Constellation":cdb[]}[] []] -> w235
          frame False {
          }
          frame True {
          }
        }
        "Constellation Map 2 Channel" <- w235
        "Constellation Map 1 Channel" <- w233
        n172 = case shown="True" w198 {
          tunnel: w197 -> [w283 w285]
          tunnel: [nan ("Graph Instantaneous BER") w285] -> w201
          tunnel: [w283 nan ("Graph Instantaneous BER")] -> w202
          frame False {
          }
          frame True {
          }
        }
        "Low-Power BER - CH0" <- w202
        "Low-Power BER - 1 Channel" <- w201
        n173 = Bundle("Graph Instantaneous BER"=w191, "Graph Instantaneous BER"=w194, "Graph Instantaneous BER"=w192) -> (w239:T9)  [unwired: 1 in]
        n174 = Equal To 0?(x="State") -> (x = 0?=w230:bool)
        "CH0 2" <- w230
        n175 = Not(x=w230) -> (.not. x?=→"CH1 2":bool)
        n176 = case shown="True" w198 {
          tunnel: w191 -> [_ w289]
          tunnel: [nan w289] -> w238
          tunnel: w239 -> [w287 _]
          tunnel: [w287 T9 {"Graph Instantaneous BER"=nan, "Graph Instantaneous BER"=nan, "Graph Instantaneous BER"=nan}] -> w240
          frame False {
          }
          frame True {
          }
        }
        "High-Power BER" <- w240
        "High-Power BER - 1 Channel" <- w238
        n177 = local write "Counter"(w223) -> ()
        n178 = local write "State"(w224) -> ()
        n179 = case shown="True" w198 {
          tunnel: w197 -> [w246 w270]
          tunnel: w191 -> [w245 w269]
          tunnel: w196 -> [w248 w268]
          tunnel: ["" w266] -> w195
          tunnel: w194 -> [w244 _]
          tunnel: w192 -> [w243 _]
          tunnel: [w242 ""] -> w193
          frame False {
            n180 = case shown="True" w248 {
              tunnel: ["" w256] -> w242
              tunnel: w246 -> [_ w254]
              tunnel: w245 -> [_ w255]
              tunnel: "Save data 2 channels" -> [_ w253]
              tunnel: w244 -> [_ w252]
              tunnel: w243 -> [_ w251]
              frame False {
              }
              frame True {
                n181 = case shown="True" w253 {
                  tunnel: ["" w262] -> w256
                  tunnel: w254 -> [_ w261]
                  tunnel: w255 -> [_ w260]
                  tunnel: w252 -> [_ w259]
                  tunnel: w251 -> [_ w258]
                  frame False {
                  }
                  frame True {
                    n182 = Build Array(w261, w260, w259, w258) -> (w264:dbl[])
                    n183 = Array To Spreadsheet String(array=w264, 3:"%.3f") -> (spreadsheet string=w262:string)  [unwired: 1 out]
                  }
                }
              }
            }
          }
          frame True {
            n184 = case shown="True" w268 {
              tunnel: ["" w275] -> w266
              tunnel: w270 -> [_ w273]
              tunnel: w269 -> [_ w274]
              tunnel: "Save data 1 channel" -> [_ w272]
              frame False {
              }
              frame True {
                n185 = case shown="True" w272 {
                  tunnel: ["" w279] -> w275
                  tunnel: w273 -> [_ w278]
                  tunnel: w274 -> [_ w277]
                  frame False {
                  }
                  frame True {
                    n186 = Build Array(w278, w277) -> (w281:dbl[])
                    n187 = Array To Spreadsheet String(array=w281, 3:"%.3f") -> (spreadsheet string=w279:string)  [unwired: 1 out]
                  }
                }
              }
            }
          }
        }
      }
    }
    n188 = Equal To 0?(x=w54) -> (x = 0?=w51:bool)
    "Boolean 6" <- w51
    n189 = And(x=w48, y=w51) -> (x .and. y?=w52:bool)
    n190 = case shown="True" w52 {
      tunnel: w62 -> [_ w96]
      tunnel: w61 -> [w86 w95]
      tunnel: w60 -> [w87 w94]
      tunnel: w59 -> [w88 w93]
      tunnel: [w86 w92] -> w58
      tunnel: [w88 w91] -> w57
      tunnel: [w87 w90] -> w56
      frame False {
      }
      frame True {
        n191 = call "is_paused.vi"("url"="url", "error in (no error)"=w94, "client handle"=w93) -> ("error out"=w98:errorcluster, "paused"=w89:bool, "client handle out"=w99:T6)  [unwired: 6 in]
        "Boolean 5" <- w89
        n192 = case shown="False" w89 {
          tunnel: w96 -> [_ w107]
          tunnel: w95 -> [w100 w109]
          tunnel: "url" -> [_ w112]
          tunnel: w98 -> [w101 w114]
          tunnel: w99 -> [w102 w113]
          tunnel: [w100 w105] -> w92
          tunnel: [w102 w104] -> w91
          tunnel: [w101 w103] -> w90
          frame True {
          }
          frame False {
            n193 = Array Size(array=w107) -> (size(s)=w106:i32)
            n194 = Index Array(array=w107, index=w109) -> (element=w115:T7)
            n195 = Increment(x=w109) -> (x+1=w108:i32)
            n196 = Quotient & Remainder(x=w108, y=w106) -> (x-y*floor(x/y)=w105:i32)  [unwired: 1 out]
            n197 = call "send_angles.vi"("url"=w112, "error in (no error)"=w114, "angles and speed"=w115, "client handle"=w113) -> ("error out"=w110:errorcluster, "client handle out"=w111:T6)  [unwired: 6 in]
            n198 = while {
              tunnel: w112 -> [w121]
              tunnel: w111 -> [w120]
              tunnel: w110 -> [w119]
              tunnel: [w117] -> w104
              tunnel: [w116] -> w103
              stop <- w118 continue-if-true
              n199 = call "is_moving.vi"("string"=w121, "error in (no error)"=w119, "client handle"=w120) -> ("error out"=w116:errorcluster, "moving"=w118:bool, "client handle out"=w117:T6)  [unwired: 6 in]
            }
          }
        }
      }
    }
    n200 = Write to Text File(file (use dialog)=w68, text=w63, error in=w67) -> (refnum out=w65:refnum<file>, error out=w66:errorcluster)  [unwired: 1 in, 1 out]
    n201 = Write to Text File(file (use dialog)=w74, text=w73, error in=w75) -> (refnum out=w76:refnum<file>, error out=w77:errorcluster)  [unwired: 1 in, 1 out]
    n202 = Write to Text File(file (use dialog)=w72, text=w64, error in=w70) -> (refnum out=w71:refnum<file>, error out=w69:errorcluster)  [unwired: 1 in, 1 out]
    "Numeric" <- w53
  }
  n203 = Close File(refnum=w28, error in=w29) -> (error out=w32:errorcluster)  [unwired: 1 out]
  n204 = Close File(refnum=w10, error in=w9) -> (error out=w16:errorcluster)  [unwired: 1 out]
  n205 = Close File(refnum=w8, error in=w7) -> (error out=w15:errorcluster)  [unwired: 1 out]
  n206 = local read "iterationsIM"() -> (→"iterationsIM":dbl)
  n207 = call <vilib>:"Simple Error Handler.vi"("error in (no error)"=w32) -> ()  [unwired: 1 in, 8 out]
  n208 = call <vilib>:"Simple Error Handler.vi"("error in (no error)"=w16) -> ()  [unwired: 1 in, 8 out]
  n209 = call <vilib>:"Simple Error Handler.vi"("error in (no error)"=w15) -> ()  [unwired: 1 in, 8 out]
  n210 = call <vilib>:"CloseHandle.vi"("client handle"=w2, "error in (no error)"=w1) -> ()  [unwired: 13 in, 1 out]
  n211 = call <instrlib>:"niUSRP Close Session.vi"("session handle"=w42, "error in (no error)"=w43) -> ()  [unwired: 13 in, 1 out]
  "No. Bits LP - CH0" <- w39
  "No. Bits - CH1" <- w39
  "No. Bits HP - CH0" <- w39
